vi "Firmware_Version_SUB_VI.vi"(5 "Message Length":i32, 6 "Firmware Response ID":u8=76, 7 "Firmware Request ID":i32=75, 8 "error in (no error)":errorcluster, 10 "remote port or service name":u16=1600, 11 "address":string="192.168.1.100") -> (0 "error out":errorcluster, 1 "PC Firmware Version":string, 2 "AC Firmware Version":string, 3 "SC Firmware Version":string)   [LabVIEW 2017]
panel:
  out "connection ID out":refnum<k5>
  out "Firmware Version":string
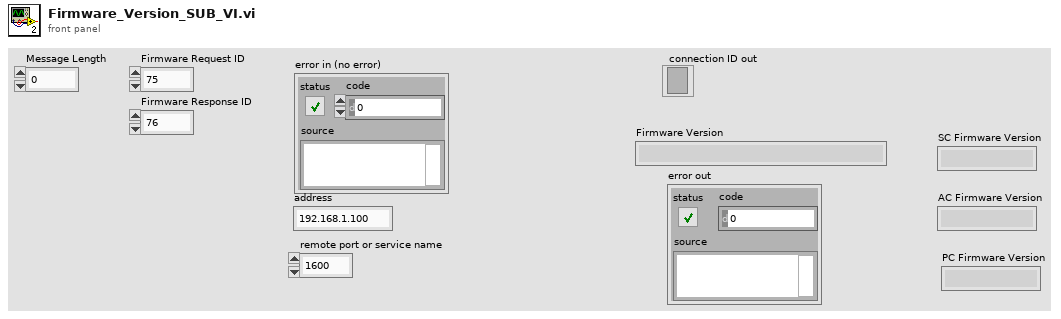
[diagram p1: front panel]
types:
  T1 = cluster{"Message Length":i32, "Firmware Request ID":i32}
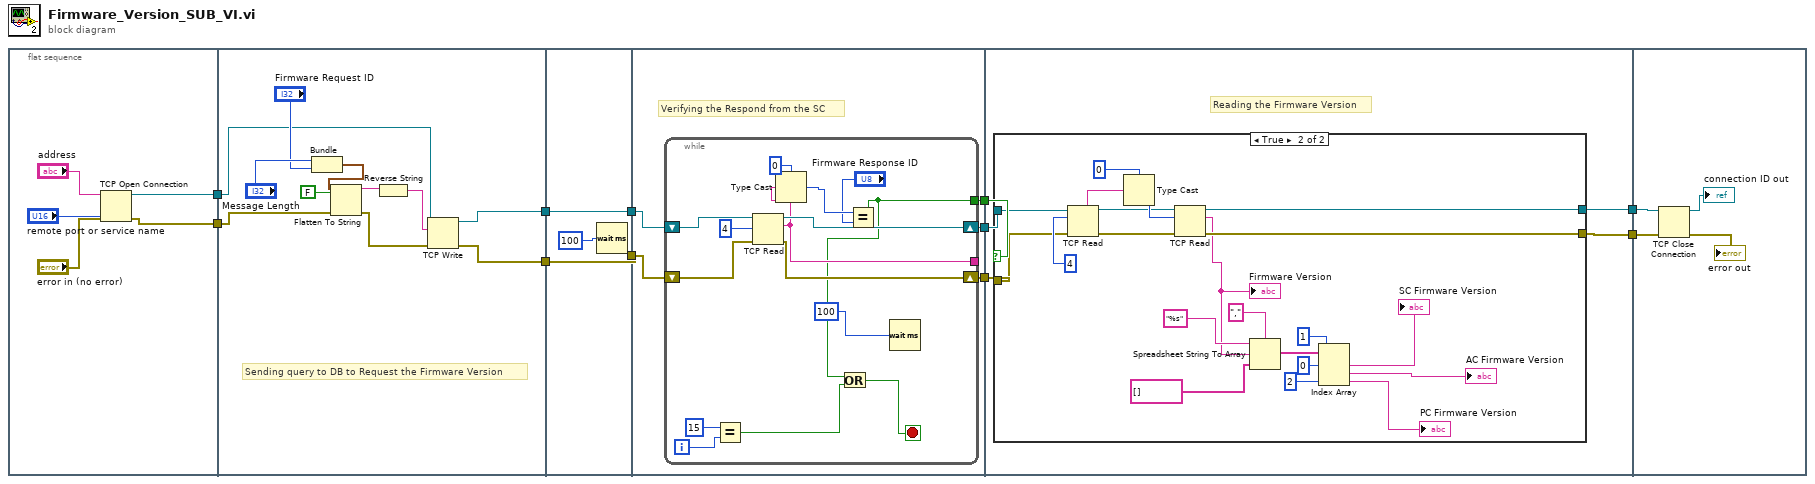
[diagram p0: block diagram]
diagram:
  n1 = flat-sequence {
    tunnel: [w13] -> w11
    tunnel: [w12] -> w10
    tunnel: w11 -> [w19]
    tunnel: w10 -> [w20]
    tunnel: [w18] -> w9
    tunnel: [w17] -> w8
    tunnel: [w29] -> w5
    tunnel: w9 -> [w29]
    tunnel: w8 -> [w28]
    tunnel: [w28] -> w4
    tunnel: w5 -> [w35]
    tunnel: w4 -> [w34]
    tunnel: [w33] -> w3
    tunnel: [w32] -> w2
    tunnel: [w31] -> w1
    tunnel: [w55] -> w7
    tunnel: [w54] -> w6
    tunnel: w3 -> [w53]
    tunnel: w2 -> [w52]
    tunnel: w1 -> [w51]
    tunnel: w7 -> [w82]
    tunnel: w6 -> [w81]
    frame #0 {
      n2 = TCP Open Connection(address="address", remote port or service name="remote port or service name", error in (no error)="error in (no error)") -> (connection ID=w12:refnum<k5>, error out=w13:errorcluster)  [unwired: 2 in]
    }
    frame #1 {
      # "Sending query to DB to Request the Firmware Version"
      n3 = Bundle("Message Length"="Message Length", "Firmware Request ID"="Firmware Request ID") -> (w21:T1)  [unwired: 1 in]
      n4 = Flatten To String(anything=w21, prepend array or string size? (T)=FALSE, error in (no error)=w19) -> (data string=w25:string, error out=w23:errorcluster)  [unwired: 1 in, 1 out]
      n5 = Reverse String(1:w25) -> (0:w24:string)
      n6 = TCP Write(connection ID=w20, data in=w24, error in (no error)=w23) -> (connection ID out=w18:refnum<k5>, error out=w17:errorcluster)  [unwired: 1 in, 1 out]
    }
    frame #2 {
      n7 = Wait (ms)(milliseconds to wait=u32 100) -> ()  [unwired: 1 out]
    }
    frame #3 {
      # "Verifying the Respond from the SC"
      n8 = while {
        tunnel: [w45] -> _
        shift-right: [w48] -> w33
        shift-left: w35 -> [w50]
        shift-right: [w46] -> w32
        shift-left: w34 -> [w49]
        tunnel: [w41] -> w31
        i -> [w39]
        stop <- w40 stop-if-true
        n9 = Equal?(x=15, y=w39) -> (x = y?=w37:bool)
        n10 = TCP Read(connection ID=w50, bytes to read=4, error in (no error)=w49) -> (connection ID out=w48:refnum<k5>, data out=w45:string, error out=w46:errorcluster)  [unwired: 2 in]
        n11 = Type Cast(type=u8 0, x=w45) -> (*(type *) &x=w43:u8)
        n12 = Equal?(x=w43, y="Firmware Response ID") -> (x = y?=w41:bool)
        n13 = Or(x=w41, y=w37) -> (x .or. y?=w40:bool)
        n14 = Wait (ms)(milliseconds to wait=i16 100) -> ()  [unwired: 1 out]
      }
    }
    frame #4 {
      # "Reading the Firmware Version"
      n15 = case shown="True" w51 {
        tunnel: [w56 w72] -> w55
        tunnel: [w57 w71] -> w54
        tunnel: w53 -> [w56 w70]
        tunnel: w52 -> [w57 w69]
        frame False {
        }
        frame True {
          n16 = TCP Read(connection ID=w70, bytes to read=4, error in (no error)=w69) -> (connection ID out=w74:refnum<k5>, data out=w77:string, error out=w73:errorcluster)  [unwired: 2 in]
          n17 = Type Cast(type=u8 0 ("bytes to read"), x=w77) -> (*(type *) &x=w75:u8)
          n18 = TCP Read(connection ID=w74, bytes to read=w75, error in (no error)=w73) -> (connection ID out=w72:refnum<k5>, data out=w58:string, error out=w71:errorcluster)  [unwired: 2 in]
          "Firmware Version" <- w58
          n19 = Spreadsheet String To Array(delimiter (Tab)=",", format string="%s", spreadsheet string=w58, array type (2D Dbl)=string[] []) -> (array=w65:string[])
          n20 = Index Array(array=w65, index #1=0 ("index"), index #2=1 ("index"), index #3=2 ("index")) -> (element #1=→"SC Firmware Version":string, element #2=→"AC Firmware Version":string, element #3=→"PC Firmware Version":string)
        }
      }
    }
    frame #5 {
      n21 = TCP Close Connection(connection ID=w82, error in (no error)=w81) -> (connection ID out=→"connection ID out":refnum<k5>, error out=→"error out":errorcluster)  [unwired: 1 in]
    }
  }
